vi "Login_Dialog_SoftFP.vi"(0 "reference in":refnum<class "Login_Dialog.lvclass">, 2 "Floating":bool, 5 "error in (no error)":errorcluster) -> (14 "reference out":refnum<class "Login_Dialog.lvclass">, 19 "error out":errorcluster)   [LabVIEW 2022 SP3, in "Login_Dialog.lvlib" / "Login_Dialog.lvclass"]
uses:
  Login_Dialog.lvclass
  Components/ViPER.lvlibp/ViPER.lvclass
  C:/Projects/Medulla/ViPER/Examples/Flux_Capacitor_Tester/Components/ViPER.lvlibp/ViPER.lvclass
panel:
  out "Logged In":bool
  out "User":string
  in  "Logout":bool
  in  "Login":bool
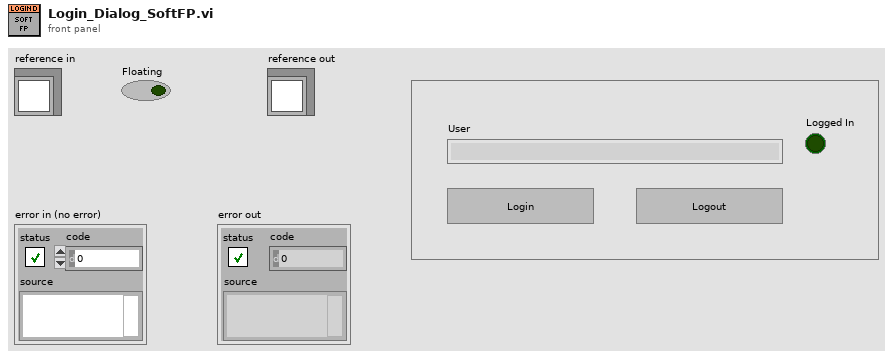
[diagram p1: front panel]
types:
  T1 = enum32{"Invalid", "Standard", "Closed", "Hidden", "Minimized", "Maximized"}
  T2 = typedef "Login_Dialog.lvlib/Login_Dialog.lvclass/ObjectAttributes.ctl" = cluster{"Config":T3, "User":string, "LoggedIn":bool, "Users":string[][]}
  T3 = typedef "Login_Dialog.lvlib/Login_Dialog.lvclass/Config.ctl" = cluster{"default":string}
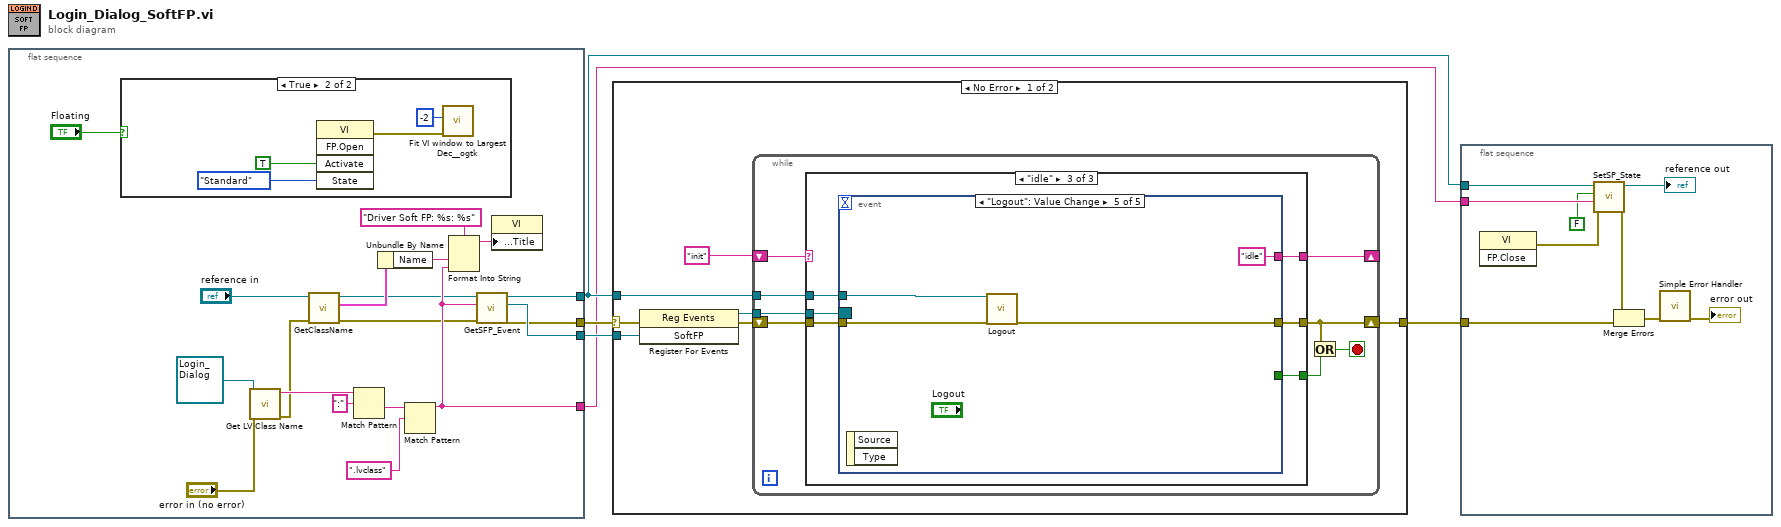
[diagram p0: block diagram]
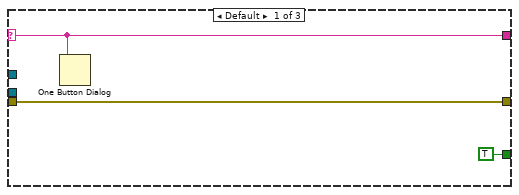
[diagram p3: hidden frame]
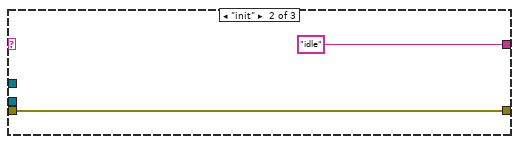
[diagram p4: hidden frame]
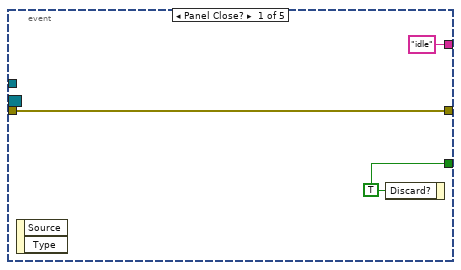
[diagram p5: hidden frame]
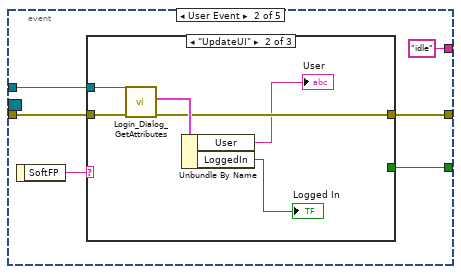
[diagram p6: hidden frame]
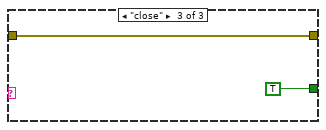
[diagram p8: hidden frame]
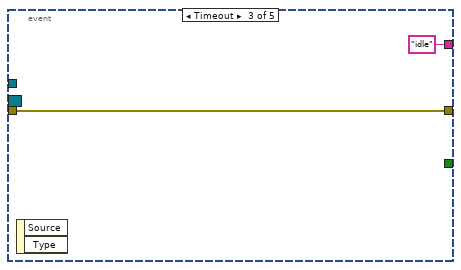
[diagram p9: hidden frame]
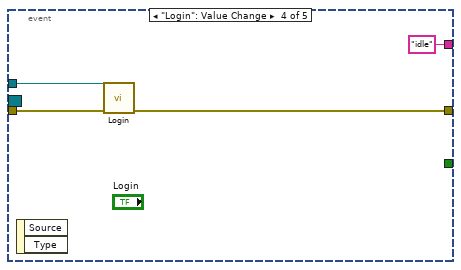
[diagram p10: hidden frame]
diagram:
  n1 = flat-sequence {
    tunnel: [w21] -> w5
    tunnel: [w20] -> w2
    tunnel: [w24] -> w3
    tunnel: [w12] -> w1
    frame #0 {
      n2 = case shown="True" "Floating" {
        frame False {
        }
        frame True {
          n3 = invoke class="VI" method="FP.Open"("Activate"=TRUE ("Activate?"), "State"=T1."Standard") -> (error out=w25:errorcluster)  [unwired: 3 in, 4 out]
          n4 = call <userlib>:"Fit VI window to Largest Dec__ogtk.vi"("error in (no error)"=w25, "border spacing (2 px)"=-2) -> ()  [unwired: 4 in, 2 out]
        }
      }
      n5 = call <vilib>:"Get LV Class Name.vi"("error in (no error)"="error in (no error)", "object"=refnum<class "Login_Dialog.lvclass"> refnum ("reference")) -> ("error out"=w11:errorcluster, "class name"=w17:string)  [unwired: 8 in]
      n6 = call "GetClassName.vi"("error in (no error)"=w11, "reference in"="reference in") -> ("error out"=w10:errorcluster, "Details"=w9:cluster{"Name":string, "Class":string}, "reference out"=w7:refnum<class "Login_Dialog.lvclass">)  [unwired: 7 in]
      n7 = Match Pattern(string=w17, regular expression=":") -> (after substring=w15:string)  [unwired: 1 in, 3 out]
      n8 = Unbundle By Name(w9) -> ("Name"=w19:string)
      n9 = Match Pattern(string=w15, regular expression=".lvclass") -> (before substring=w12:string)  [unwired: 1 in, 3 out]
      n10 = Format Into String(format string="Driver Soft FP: %s: %s", w19, w12) -> (resulting string=w23:string)  [unwired: 2 in, 1 out]
      n11 = call-dynamic "GetSFP_Event.vi"("error in (no error)"=w10, "Ancestor"=w12, "reference in"=w7) -> ("error out"=w21:errorcluster, "SoftFP"=w24:refnum<user-event>, "reference out"=w20:refnum<class "Login_Dialog.lvclass">)  [unwired: 6 in]
      n12 = property class="VI"("Front Panel.Title"=w23) -> ()  [unwired: 2 in, 2 out]
    }
  }
  n13 = case shown="No Error" w5 {
    selector: w5 -> [w33 w83]
    tunnel: [w29 w83] -> w4
    tunnel: w2 -> [w30 _]
    tunnel: w3 -> [w35 _]
    frame No Error {
      n14 = register-events(error in=w33, w35) -> (reference out=w34:refnum<event-registration>, error out=w32:errorcluster)  [unwired: 1 in]
      n15 = while {
        shift-right: [w40] -> w29
        shift-left: w32 -> [w43]
        tunnel: w34 -> [w42]
        tunnel: w30 -> [w41]
        shift-right: [w36] -> _
        shift-left: "init" -> [w37]
        stop <- w39 stop-if-true
        n16 = case shown="\"idle\"" w37 {
          selector: w37 -> [w44 _ _]
          tunnel: w43 -> [w45 w47 w54]
          tunnel: w42 -> [_ _ w53]
          tunnel: w41 -> [_ _ w52]
          tunnel: [w45 w47 w51] -> w40
          tunnel: [TRUE ("Discard?") _ w50] -> w38
          tunnel: [w44 "idle" w49] -> w36
          frame Default {
            n17 = One Button Dialog(message=w44) -> ()  [unwired: 1 in, 1 out]
          }
          frame "init" {
          }
          frame "idle" {
            n18 = event shown="[4] \"Logout\": Value Change" {
              selector: w53 -> [_ _ _ _ _]
              dyn-events: _ -> [_ _ _ _ _]
              timeout: _ -> [_ _ _ _ _]
              tunnel: w54 -> [w57 w63 w74 w77 w82]
              tunnel: [w57 w61 w74 w76 w80] -> w51
              tunnel: [w56 w60 _ _ _] -> w50
              tunnel: w52 -> [_ w58 _ w78 w81]
              tunnel: ["idle" "idle" "idle" "idle" "idle"] -> w49
              event Panel Close? {
                w56 = TRUE ("Discard?")
                n19 = event-data() -> ()  [unwired: 1 in, 2 out]
                n20 = event-data("Discard?"=w56) -> ()  [unwired: 1 in, 1 out]
              }
              event User Event {
                n21 = event-data() -> ("SoftFP"=w62:string)  [unwired: 1 in]
                n22 = case shown="\"UpdateUI\"" w62 {
                  tunnel: w63 -> [w64 w70 w72]
                  tunnel: [w64 w67 w72] -> w61
                  tunnel: [_ _ TRUE ("Discard?")] -> w60
                  tunnel: w58 -> [_ w69 _]
                  frame Default {
                  }
                  frame "UpdateUI" {
                    n23 = call "Login_Dialog_GetAttributes.vi"("error in (no error)"=w70, "reference in"=w69) -> ("error out"=w67:errorcluster, "Data"=w68:T2)  [unwired: 6 in, 2 out]
                    n24 = Unbundle By Name(w68) -> ("User"=→"User":string, "LoggedIn"=→"Logged In":bool)
                  }
                  frame "close" {
                  }
                }
              }
              event Timeout {
                n25 = event-data() -> ()  [unwired: 1 in, 2 out]
              }
              event "Login": Value Change {
                n26 = event-data() -> ()  [unwired: 1 in, 2 out]
                n27 = call-dynamic "Login.vi"("reference in"=w78, "error in (no error)"=w77) -> ("error out"=w76:errorcluster)  [unwired: 7 in, 6 out]
              }
              event "Logout": Value Change {
                n28 = event-data() -> ()  [unwired: 1 in, 2 out]
                n29 = call-dynamic "Logout.vi"("reference in"=w81, "error in (no error)"=w82) -> ("error out"=w80:errorcluster)  [unwired: 16 in, 1 out]
              }
            }
          }
        }
        n30 = Or(x=w40, y=w38) -> (x .or. y?=w39:bool)
      }
    }
    frame Error {
    }
  }
  n31 = flat-sequence {
    tunnel: w4 -> [w90]
    tunnel: w2 -> [w85]
    tunnel: w1 -> [w87]
    frame #0 {
      n32 = invoke class="VI" method="FP.Close"() -> (error out=w89:errorcluster)  [unwired: 3 in, 2 out]
      n33 = call "SetSP_State.vi"("error in (no error)"=w89, "Ancestor"=w87, "SP Open"=FALSE, "reference in"=w85) -> ("error out"=w88:errorcluster, "reference out"=→"reference out":refnum<class "Login_Dialog.lvclass">)  [unwired: 6 in]
      n34 = Merge Errors(w88, w90) -> (w92:errorcluster)
      n35 = call <vilib>:"Simple Error Handler.vi"("error in (no error)"=w92) -> ("error out"=→"error out":errorcluster)  [unwired: 4 in, 4 out]
    }
  }
